vi "Compare and wr MODBUS regs (SubVI).vi"(0 "Modbus Master in":refnum<class "Modbus Master.lvclass">, 2 "control":u16, 5 "modbus read arr in":u16[](array[numeric]), 7 "arr el. index":u16, 11 "error in (no error)":errorcluster, 13 "reg address":u16) -> (4 "Modbus Master out":refnum<class "Modbus Master.lvclass">, 6 "modbus read arr  out":u16[](array[numeric]), 15 "error out":errorcluster)   [LabVIEW 2015]
uses:
  <vilib>/NI/Modbus Library/API/Master/Modbus Master.lvclass
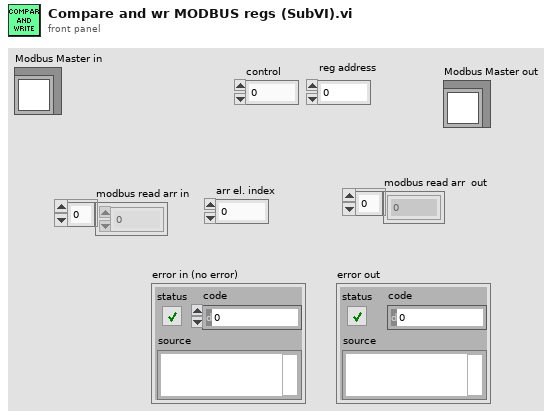
[diagram p1: front panel]
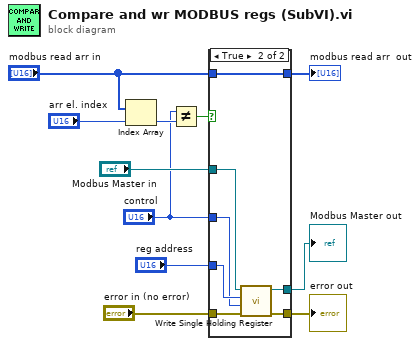
[diagram p0: block diagram]
diagram:
  n1 = Index Array(array="modbus read arr in", index="arr el. index") -> (element=w5:u16)
  n2 = Not Equal?(x="control", y=w5) -> (x != y?=w11:bool)
  n3 = case shown="True" w11 {
    tunnel: "Modbus Master in" -> [w14 w21]
    tunnel: "error in (no error)" -> [w13 w20]
    tunnel: [w14 w19] -> w9
    tunnel: [w13 w18] -> w10
    tunnel: "reg address" -> [_ w17]
    tunnel: "modbus read arr in" -> [w12 w16]
    tunnel: [w12 w16] -> w2
    tunnel: "control" -> [_ w15]
    frame False {
    }
    frame True {
      n4 = call-dynamic "Write Single Holding Register.vi"("error in"=w20, "register to write"=w15, "address"=w17, "Modbus master in"=w21) -> ("error out"=w18:errorcluster, "Modbus master out"=w19:refnum<class "Modbus Master.lvclass">)  [unwired: 6 in]
    }
  }
  "error out" <- w10
  "Modbus Master out" <- w9
  "modbus read arr  out" <- w2
